vi "Set PanelVIRefs.vi"(8 "error in (no error)":errorcluster caption="错误输入（无错误）", 11 "PanelDataNode 输入":refnum<class "PanelDataNode.lvclass"> caption="DNL_LabVIEW Object in") -> (0 "error out":errorcluster caption="错误输出", 1 "VerticalPanel":refnum<vi>, 2 "HorizontalPanel":refnum<vi>, 3 "PanelDataNode 输出":refnum<class "PanelDataNode.lvclass"> caption="DNL_LabVIEW Object out")   [LabVIEW 2016, in "PanelDataNode.lvclass"]
uses:
  PanelDataNode.lvclass
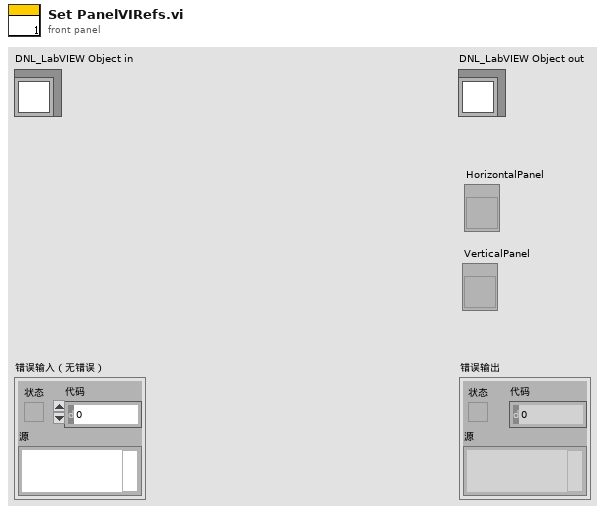
[diagram p1: front panel]
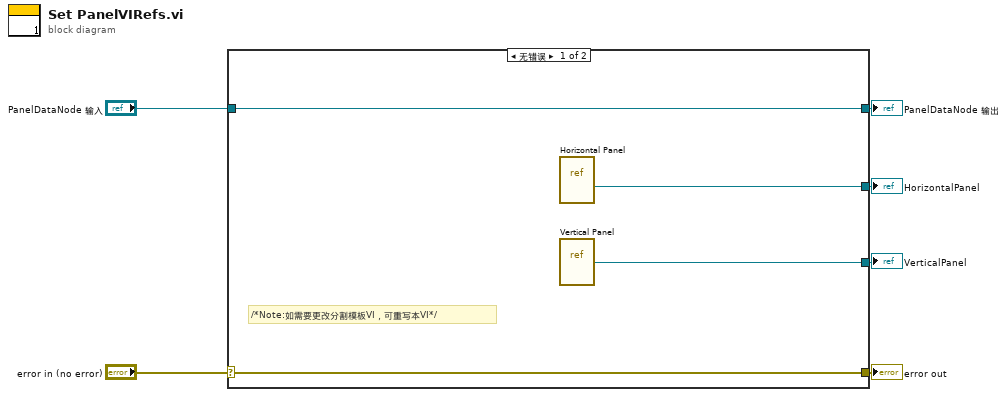
[diagram p0: block diagram]
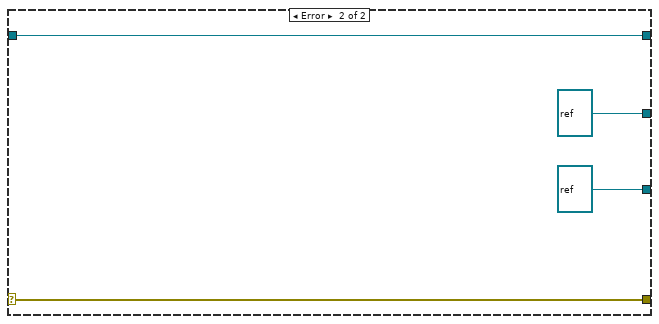
[diagram p2: hidden frame]
diagram:
  n1 = case shown="无错误" "error in (no error)" {
    selector: "error in (no error)" -> [w10 w14]
    tunnel: [w10 w14] -> w5
    tunnel: [w7 w13] -> w3
    tunnel: "PanelDataNode 输入" -> [w7 w13]
    tunnel: [w9 refnum<vi> refnum] -> w2
    tunnel: [w8 refnum<vi> refnum] -> w1
    frame No Error {
      # "/*Note:如需要更改分割模板VI，可重写本VI*/"
      n2 = vi-ref "Horizontal Panel.vi"() -> (w9:refnum<vi>)
      n3 = vi-ref "Vertical Panel.vi"() -> (w8:refnum<vi>)
    }
    frame Error {
    }
  }
  "error out" <- w5
  "PanelDataNode 输出" <- w3
  "HorizontalPanel" <- w2
  "VerticalPanel" <- w1
